vi "conect and open A.vi"(0 "设置":T1, 1 "Card ID":string) -> (5 "Output Handle":cluster{"Session":u32, "Card number":u32}, 6 "find?":bool, 7 "error out":errorcluster {"code" format="%.0x"})   [LabVIEW 2018]
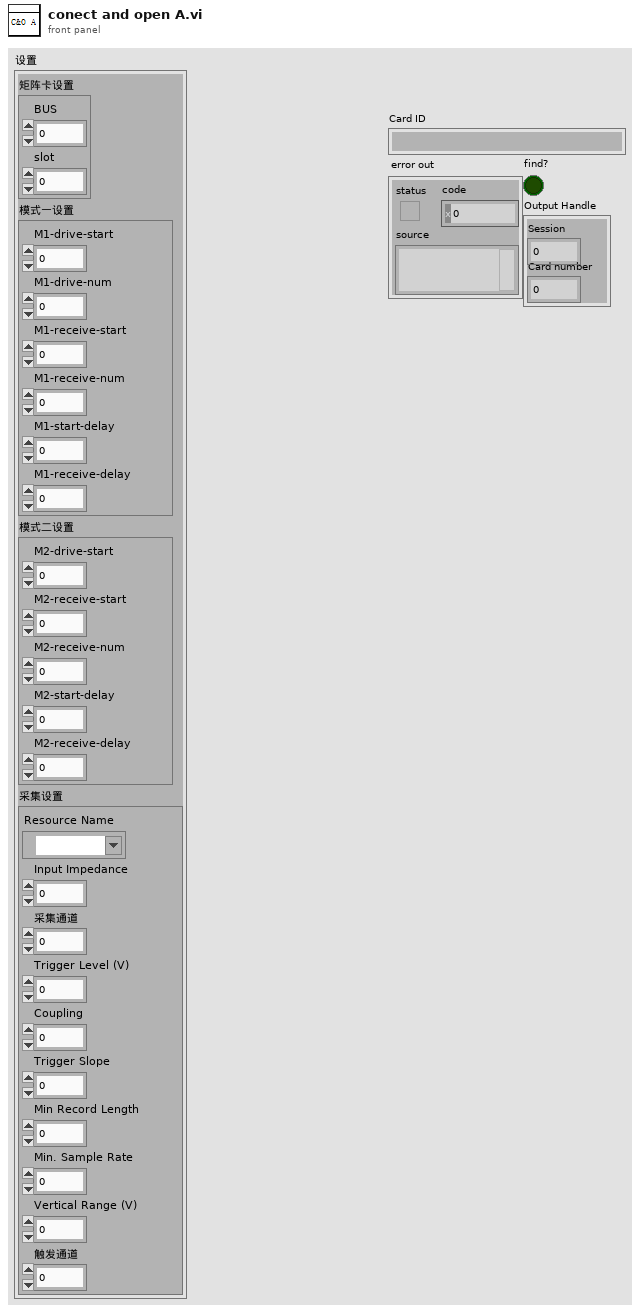
[diagram p1: front panel]
types:
  T1 = cluster{"矩阵卡设置":cluster{"BUS":u32, "slot":u32}, "模式一设置":cluster{"M1-drive-start":u32, "M1-drive-num":u32, "M1-receive-start":u32, "M1-receive-num":u32, "M1-start-delay":u32, "M1-receive-delay":u32}, "模式二设置":cluster{"M2-drive-start":u32, "M2-receive-start":u32, "M2-receive-num":u32, "M2-start-delay":u32, "M2-receive-delay":u32}, "采集设置":cluster{"Resource Name":refnum<k15>, "Input Impedance":u32, "采集通道":i32, "Trigger Level (V)":dbl, "Coupling":u16, "Trigger Slope":i32, "Min Record Length":i32, "Min. Sample Rate":dbl, "Vertical Range (V)":dbl, "触发通道":i32}}
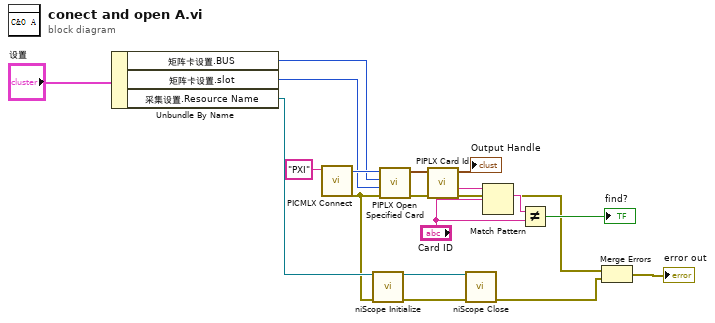
[diagram p0: block diagram]
diagram:
  n1 = Unbundle By Name("设置") -> ("矩阵卡设置.BUS"=w10:u32, "矩阵卡设置.slot"=w9:u32, "采集设置.Resource Name"=w8:refnum<k15>)
  n2 = call <instrlib>:"PICMLX Connect.vi"("Remote Machine"="PXI") -> ("error out"=w5:errorcluster, "Session"=w19:u32)  [unwired: 8 in]
  n3 = call <instrlib>:"niScope Initialize.vi"("resource name"=w8, "error in"=w5) -> ("instrument handle"=w7:refnum<k15>, "error out"=w6:errorcluster)  [unwired: 12 in]
  n4 = call <instrlib>:"PIPLX Open Specified Card.vi"("error in"=w5, "Slot"=w9, "Bus"=w10, "Session"=w19) -> ("error out"=w18:errorcluster, "Output Handle"=w17:cluster{"Session":u32, "Card number":u32})  [unwired: 6 in]
  n5 = call <instrlib>:"PIPLX Card Id.vi"("error in"=w18, "Input Handle"=w17) -> ("error out"=w4:errorcluster, "Card ID"=w16:string, "Output Handle"=→"Output Handle":cluster{"Session":u32, "Card number":u32})  [unwired: 7 in]
  n6 = call <instrlib>:"niScope Close.vi"("instrument handle"=w7, "error in"=w6) -> ("error out"=w3:errorcluster)  [unwired: 13 in]
  n7 = Match Pattern(string=w16, regular expression="Card ID") -> (match substring=w15:string)  [unwired: 1 in, 3 out]
  n8 = Not Equal?(x=w15, y="Card ID") -> (x != y?=→"find?":bool)
  n9 = Merge Errors(w4, w3) -> (→"error out":errorcluster)
